vi "ReadArea.vi"() -> ()   [LabVIEW 2016]
uses:
  lib/Snap7.lvlib
panel:
  out "?":string
  out "ASCII Data":string
  out "Hex Data":string
  out "Running":bool
  out "Status":string="No Error"
  in  "Word Length":i32(ring)=2 items=["Bit"=1, "Byte"=2, "Word"=4, "DWord"=6, "Real"=8, "Counter"=28, "Timer"=29]
  in  "Area":i32(ring)=132 items=["Inputs (EB)"=129, "Output (AB)"=130, "Bit Memory (M)"=131, "Data (DB)"=132, "Counters (Z)"=28, "Timers (T)"=29]
  in  "Amount":i32=16
  in  "Start":i32
  in  "DB Number":i32=1
  out "Data":u8[](array[numeric])
  in  "?":bool
  in  "Slot":i32=2
  in  "Rack":i32
  in  "Address IP":string="192.168.1.12"
  # "Data Read"
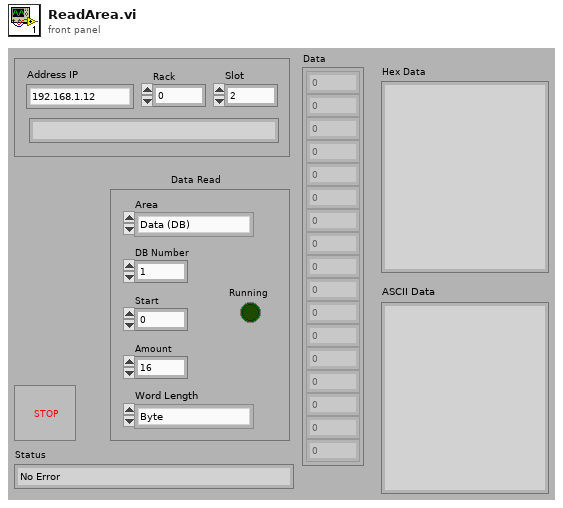
[diagram p1: front panel]
types:
  T1 = enum16{"big-endian, network order", "native, host order", "little-endian"}
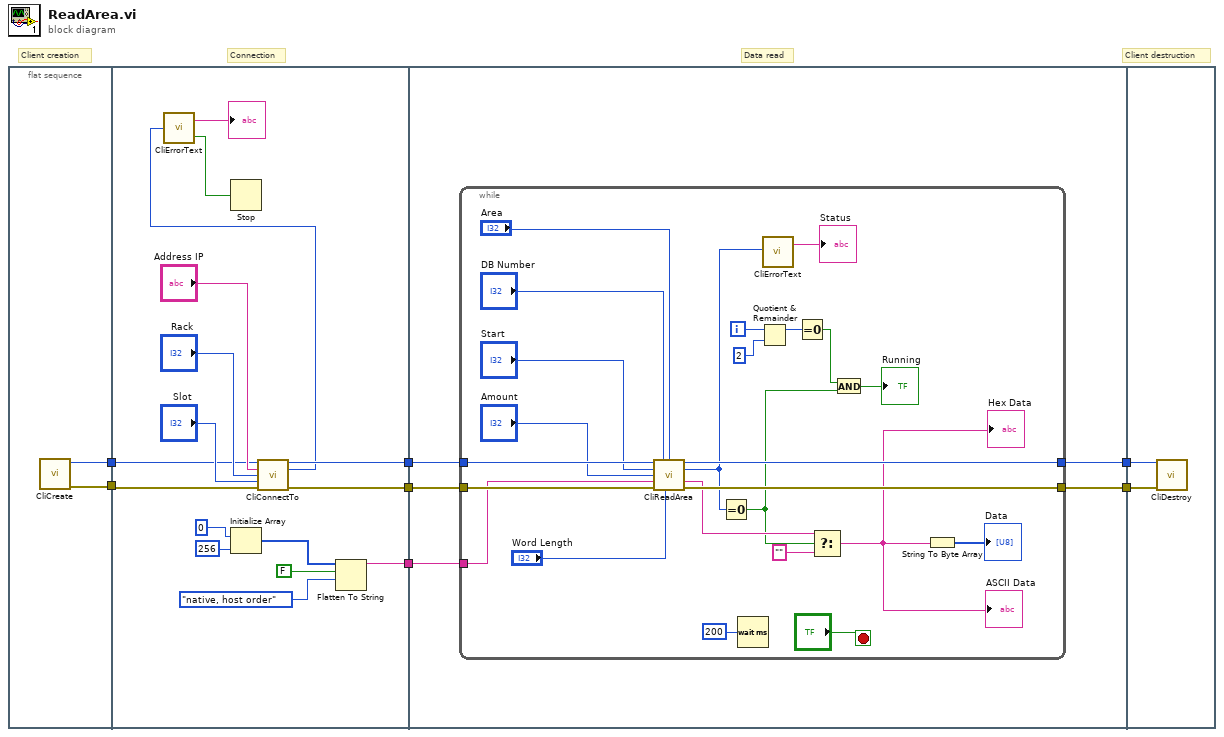
[diagram p0: block diagram]
diagram:
  # "Client destruction"
  # "Data read"
  # "Connection"
  # "Client creation"
  n1 = flat-sequence {
    tunnel: [w9] -> w4
    tunnel: [w8] -> w3
    tunnel: [w20] -> w7
    tunnel: [w13] -> w6
    tunnel: [w19] -> w5
    tunnel: w4 -> [w15]
    tunnel: w3 -> [w14]
    tunnel: w7 -> [w30]
    tunnel: w6 -> [w29]
    tunnel: w5 -> [w28]
    tunnel: [w27] -> w2
    tunnel: [w26] -> w1
    tunnel: w2 -> [w56]
    tunnel: w1 -> [w55]
    frame #0 {
      n2 = call "CliCreate.vi"() -> ("ref out"=w9:u64, "error out"=w8:errorcluster)  [unwired: 14 in]
    }
    frame #1 {
      n3 = Initialize Array(u8 0, 256) -> (w23:u8[])
      n4 = call "CliConnectTo.vi"("ref in"=w15, "Address"="Address IP", "Rack"="Rack", "Slot"="Slot", "error in (no error)"=w14) -> ("ref out"=w13:u64, "Result"=w10:i32, "error out"=w20:errorcluster)  [unwired: 8 in]
      n5 = call "CliErrorText.vi"("ErrNo"=w10) -> ("Error"=w11:bool, "ErrMessage"=→"?":string)
      n6 = Stop(stop? (T)=w11) -> ()
      n7 = Flatten To String(anything=w23, prepend array or string size? (T)=FALSE, byte order (0:big-endian, network order)=T1."native, host order") -> (data string=w19:string)  [unwired: 1 in, 2 out]
    }
    frame #2 {
      n8 = while {
        tunnel: w30 -> [w52]
        tunnel: w29 -> [w51]
        tunnel: w28 -> [w50]
        tunnel: [w44] -> w27
        tunnel: [w43] -> w26
        i -> [w41]
        stop <- "?" stop-if-true
        n9 = call "CliReadArea.vi"("ref in"=w51, "DB Number"="DB Number", "Area"="Area", "Start"="Start", "Amount"="Amount", "data in"=w50, "error in (no error)"=w52, "Word Length"="Word Length") -> ("ref out"=w44:u64, "Result"=w42:i32, "data out"=w35:string, "error out"=w43:errorcluster)  [unwired: 4 in]
        n10 = Equal To 0?(x=w42) -> (x = 0?=w34:bool)
        n11 = Wait (ms)(milliseconds to wait=u32 200 ("Loop Delay (ms)")) -> ()  [unwired: 1 out]
        n12 = Quotient & Remainder(x=w41, y=2) -> (x-y*floor(x/y)=w39:i32)  [unwired: 1 out]
        n13 = call "CliErrorText.vi"("ErrNo"=w42) -> ("ErrMessage"=→"Status":string)  [unwired: 1 out]
        n14 = Equal To 0?(x=w39) -> (x = 0?=w38:bool)
        n15 = Select(t=w35, s=w34, f="") -> (s? t:f=w32:string)
        "ASCII Data" <- w32
        "Hex Data" <- w32
        n16 = And(x=w38, y=w34) -> (x .and. y?=→"Running":bool)
        n17 = String To Byte Array(string=w32) -> (unsigned byte array=→"Data":u8[])
      }
    }
    frame #3 {
      n18 = call "CliDestroy.vi"("ref in"=w56, "error in (no error)"=w55) -> ()  [unwired: 13 in, 1 out]
    }
  }
